vi "Autonomous Independent.vi"() -> ()   [LabVIEW 2013]
doc: "This VI is called when autonomous begins, and will automatically be terminated when autonomous ends. You can carry out timed or sensor driven robot movement independently without needing to return to the caller."
uses:
  Robot Global Data.vi
panel:
  in  "Forward 3 (ms)":u32=1000
  in  "Forward 2 (ms)":u32=800
  in  "Back Duration (ms)":u32=750
  in  "Forward 1 (ms)":u32=250
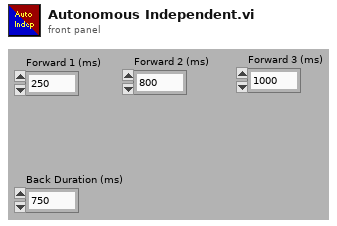
[diagram p1: front panel]
types:
  T1 = enum16{"Hold", "Pick Up", "Catch", "Aim", "Shoot"}
  T2 = typedef "WPI_DriverStationMatch Info.ctl" = cluster{"Autonomous Elapsed Seconds":dbl, "TeleOp Elapsed Seconds":dbl, "Disabled Elapsed Seconds":dbl, "Visited Autonomous":bool, "Visited TeleOp":bool, "Visited Disabled":bool, "Autonomous Settings":cluster{"Autonomous Style":enum16{"Iterative", "Independent"}, "VI Refnum":refnum<vi>}}
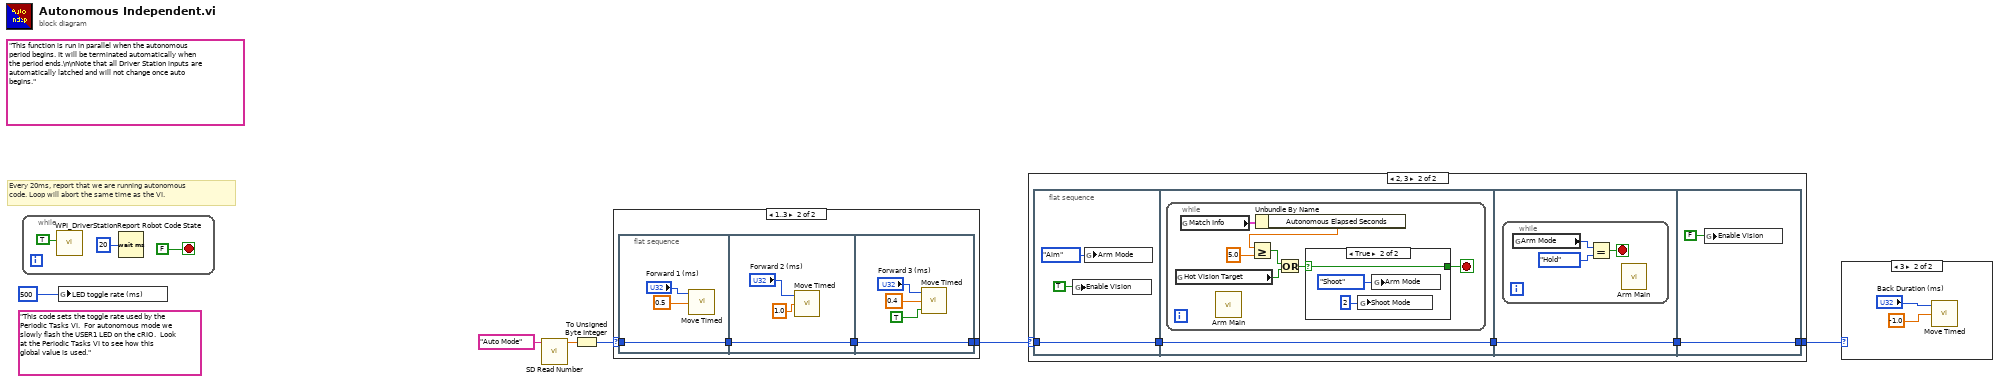
[diagram p0: block diagram]
diagram:
  (unwired) "This code sets the toggle rate used by the Periodic Tasks VI.  For autonomous mode we slowly flash the USER1 LED on the cRIO.  Look at the Periodic Tasks VI to see how this global value is used."
  (unwired) "This function is run in parallel when the autonomous period begins. It will be terminated automatically when the period ends.\n\nNote that all Driver Station inputs are automatically latched and will not change once auto begins."
  # "Every 20ms, report that we are running autonomous\ncode. Loop will abort the same time as the VI."
  n1 = while {
    stop <- FALSE stop-if-true
    n2 = call <vilib>:"WPI_DriverStationReport Robot Code State.vi"("Autonomous"=TRUE) -> ()  [unwired: 10 in, 1 out]
    n3 = Wait (ms)(milliseconds to wait=u32 20) -> ()  [unwired: 1 out]
  }
  n4 = global write "Robot Global Data.vi" "LED toggle rate (ms)"(u32 500 ("LED ms toggle rate")) -> ()
  n5 = call <vilib>:"SD Read Number.vi"("Name"="Auto Mode") -> ("Numeric"=w4:dbl)  [unwired: 8 in, 2 out]
  n6 = To Unsigned Byte Integer(number=w4) -> (unsigned 8bit integer=w1:u8)
  n7 = case shown="1..3" w1 {
    selector: w1 -> [w10 w11]
    tunnel: [w10 w14] -> w2
    frame 0, Default {
    }
    frame 1..3 {
      n8 = flat-sequence {
        tunnel: [w15] -> w12
        tunnel: w11 -> [w15]
        tunnel: [w18] -> w13
        tunnel: w12 -> [w18]
        tunnel: [w22] -> w14
        tunnel: w13 -> [w22]
        frame #0 {
          n9 = call "Move Timed.vi"("Move Speed"=0.5, "Move Duration (ms)"="Forward 1 (ms)") -> ()  [unwired: 2 in]
        }
        frame #1 {
          n10 = call "Move Timed.vi"("Move Speed"=1.0, "Move Duration (ms)"="Forward 2 (ms)") -> ()  [unwired: 2 in]
        }
        frame #2 {
          n11 = call "Move Timed.vi"("Break on Stop"=TRUE, "Move Speed"=0.4, "Move Duration (ms)"="Forward 3 (ms)") -> ()  [unwired: 1 in]
        }
      }
    }
  }
  n12 = case shown="2, 3" w2 {
    selector: w2 -> [w25 w26]
    tunnel: [w25 w30] -> w3
    frame 0, Default {
    }
    frame 2, 3 {
      n13 = flat-sequence {
        tunnel: [w31] -> w27
        tunnel: w26 -> [w31]
        tunnel: [w34] -> w28
        tunnel: w27 -> [w34]
        tunnel: [w46] -> w29
        tunnel: w28 -> [w46]
        tunnel: [w50] -> w30
        tunnel: w29 -> [w50]
        frame #0 {
          n14 = global write "Robot Global Data.vi" "Enable Vision"(TRUE ("Enable Vision")) -> ()
          n15 = global write "Robot Global Data.vi" "Arm Mode"(T1."Aim" ("Arm Mode")) -> ()
        }
        frame #1 {
          n16 = while {
            stop <- w35 stop-if-true
            n17 = global read "Robot Global Data.vi" "Hot Vision Target"() -> (w37:bool)
            n18 = global read "Robot Global Data.vi" "Match Info"() -> (w41:T2)
            n19 = call "Arm Main.vi"() -> ()  [unwired: 1 in]
            n20 = Unbundle By Name(w41) -> ("Autonomous Elapsed Seconds"=w39:dbl)
            n21 = Greater Or Equal?(x=w39, y=5.0) -> (x >= y?=w38:bool)
            n22 = Or(x=w38, y=w37) -> (x .or. y?=w36:bool)
            n23 = case shown="True" w36 {
              selector: w36 -> [w42 w43]
              tunnel: [w42 w43] -> w35
              frame False {
              }
              frame True {
                n24 = global write "Robot Global Data.vi" "Shoot Mode"(i8 2 ("Shoot Mode")) -> ()
                n25 = global write "Robot Global Data.vi" "Arm Mode"(T1."Shoot" ("Arm Mode")) -> ()
              }
            }
          }
        }
        frame #2 {
          n26 = while {
            stop <- w47 stop-if-true
            n27 = global read "Robot Global Data.vi" "Arm Mode"() -> (w49:T1)
            n28 = Equal?(x=w49, y=T1."Hold" ("Arm Mode")) -> (x = y?=w47:bool)
            n29 = call "Arm Main.vi"() -> ()  [unwired: 1 in]
          }
        }
        frame #3 {
          n30 = global write "Robot Global Data.vi" "Enable Vision"(FALSE ("Enable Vision")) -> ()
        }
      }
    }
  }
  n31 = case shown="3" w3 {
    frame 0, Default {
    }
    frame 3 {
      n32 = call "Move Timed.vi"("Move Speed"=-1.0, "Move Duration (ms)"="Back Duration (ms)") -> ()  [unwired: 2 in]
    }
  }
